vi "Dave_app.vi"() -> ()   [LabVIEW 2015]
uses:
  <vilib>/Utility/file.llb/Write Delimited Spreadsheet (DBL).vi
panel:
  out "Set Value":dbl format="%_6f"
  out "Pcc(uW)":dbl
  out "Vcc(V)":dbl
  out "Icc(uA)":dbl
  in  "Stop":bool
  in  "Export To CSV":bool
  out "Data 2":cluster{dbl[], dbl[]}[](array[cluster])
  out "XY Graph 2":cluster{dbl[], dbl[]}[](graph)
  in  "Voltage Stop (uV)":dbl=0.02
  out "Stop(uA)":dbl
  in  "Load From File":bool
  in  "Save To File":bool
  in  "Clear Last Value":bool
  in  "Clear Graph":bool
  in  "Get Vol":bool
  in  "stop":bool
  out "Data":cluster{dbl[], dbl[]}[](array[cluster])
  in  "VISA resource name":refnum<visa-resource-name>="VAL_N6705B"
  out "XY Graph":cluster{dbl[], dbl[]}[](graph)
  in  "Maker 2 (s)":u16=7
  out "N":u16
  in  "Step(uA)":dbl=10.0
  in  "Start (uA)":dbl min=-1e-05 max=0.0
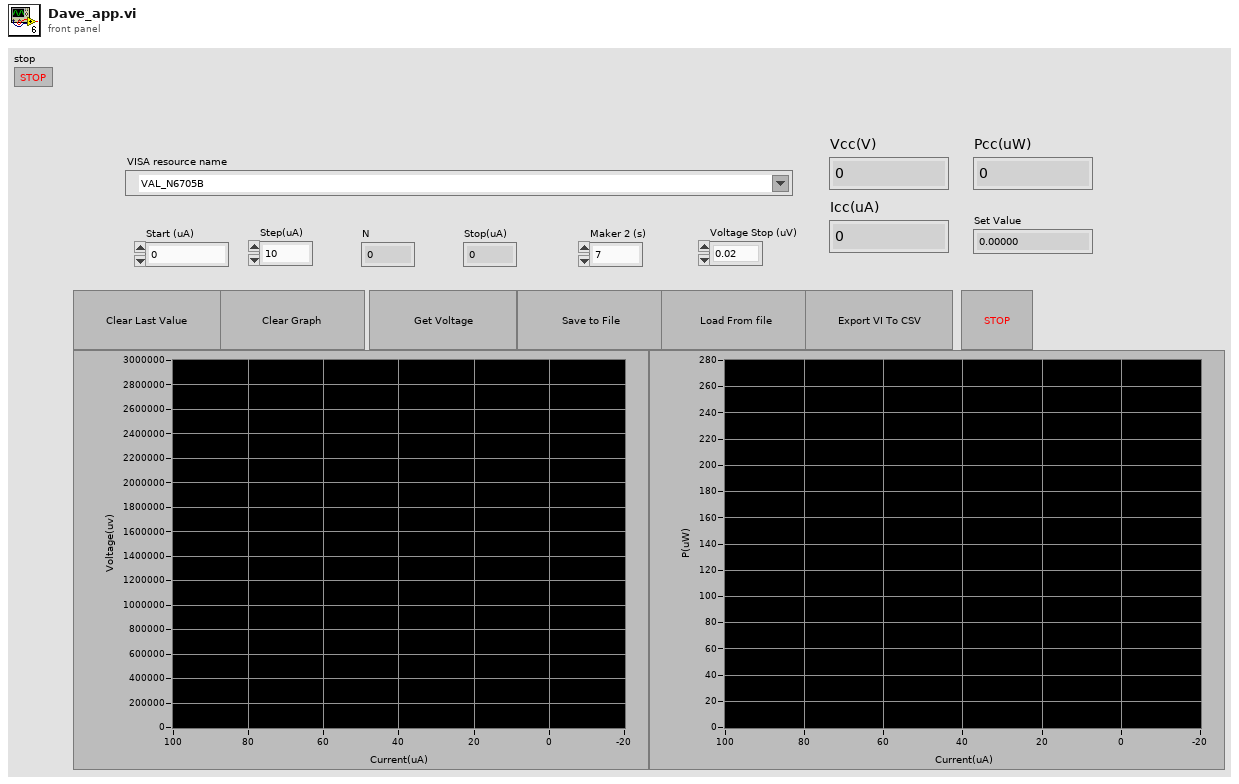
[diagram p1: front panel]
types:
  T1 = enum16{"open", "replace", "create", "open or create", "replace or create", "replace or create with confirmation"}
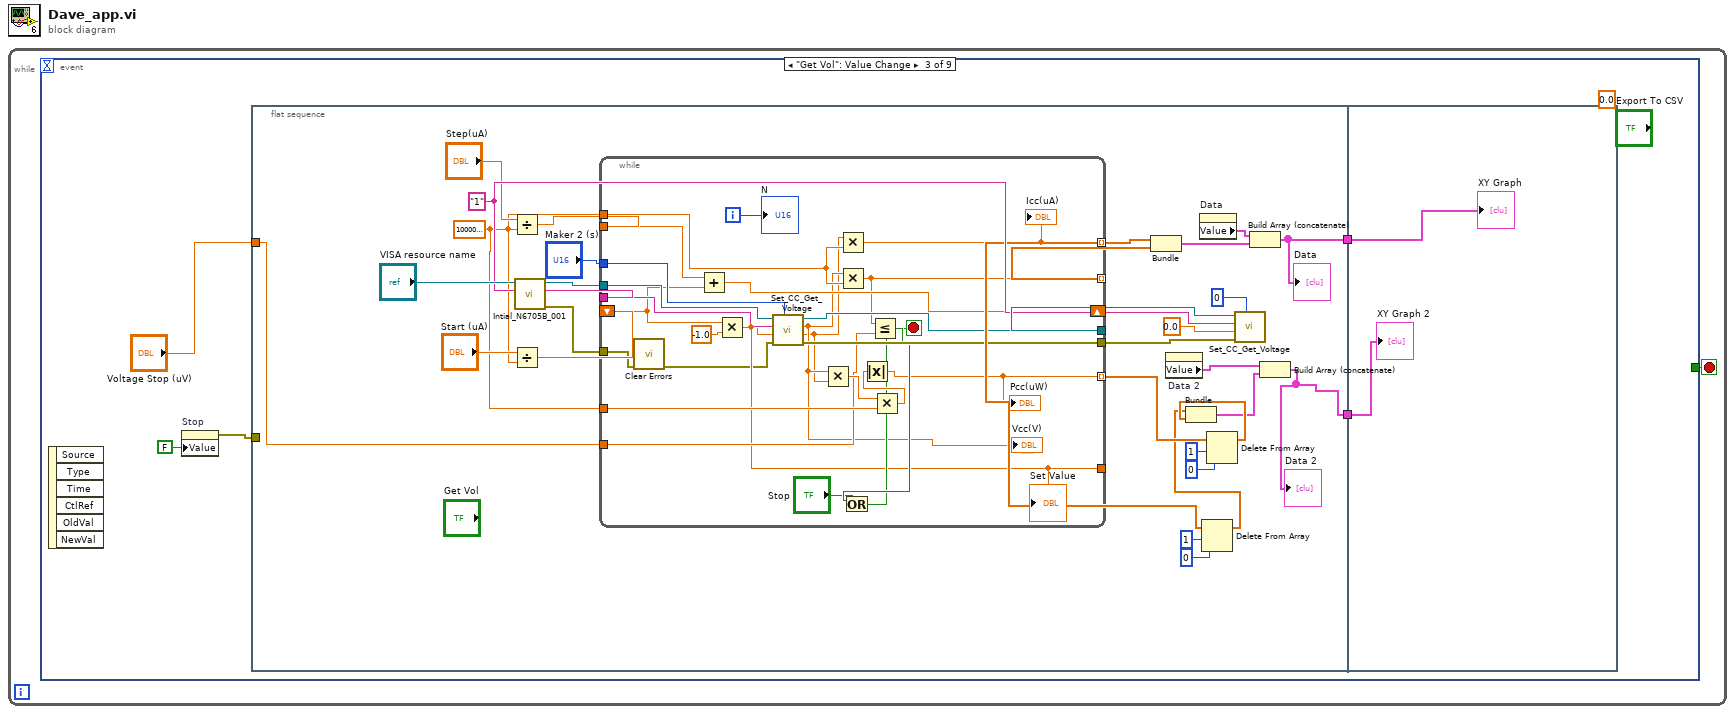
[diagram p0: block diagram]
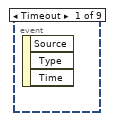
[diagram p2: hidden frame]
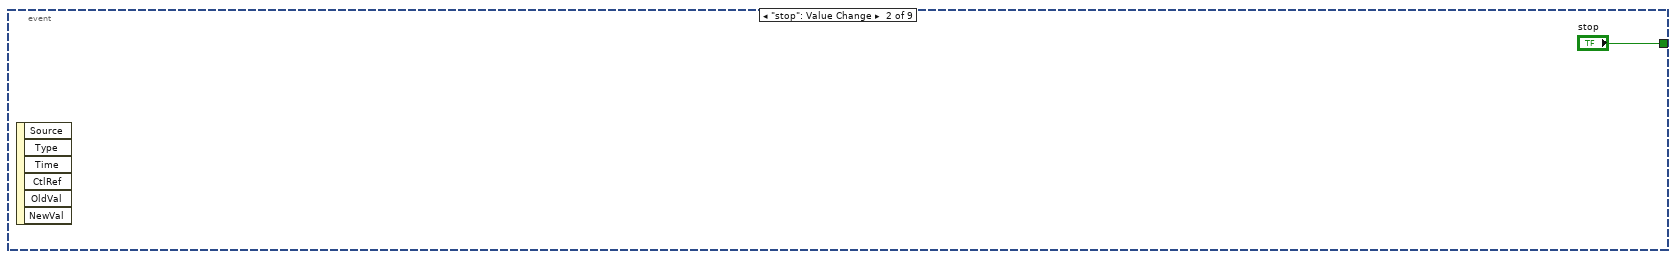
[diagram p3: hidden frame]
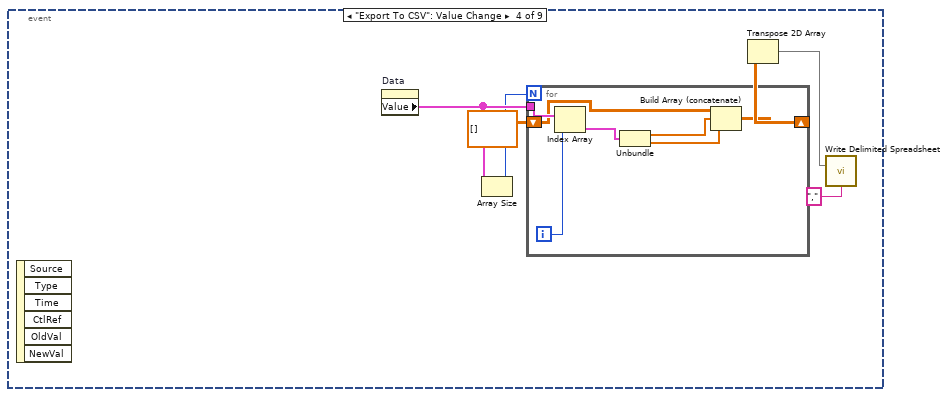
[diagram p4: hidden frame]
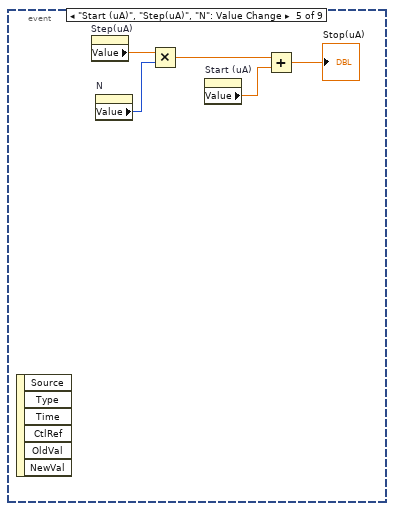
[diagram p5: hidden frame]
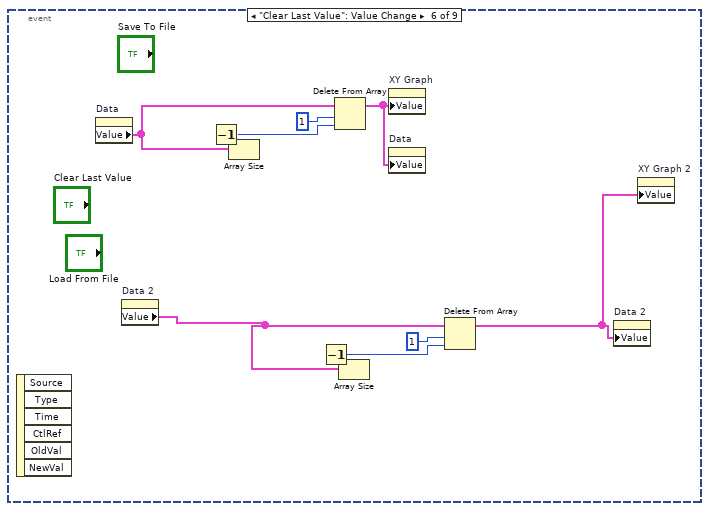
[diagram p6: hidden frame]
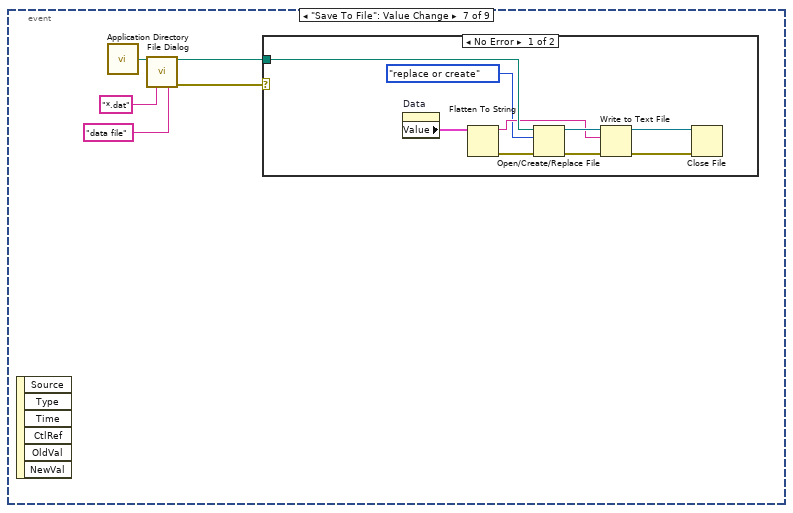
[diagram p7: hidden frame]
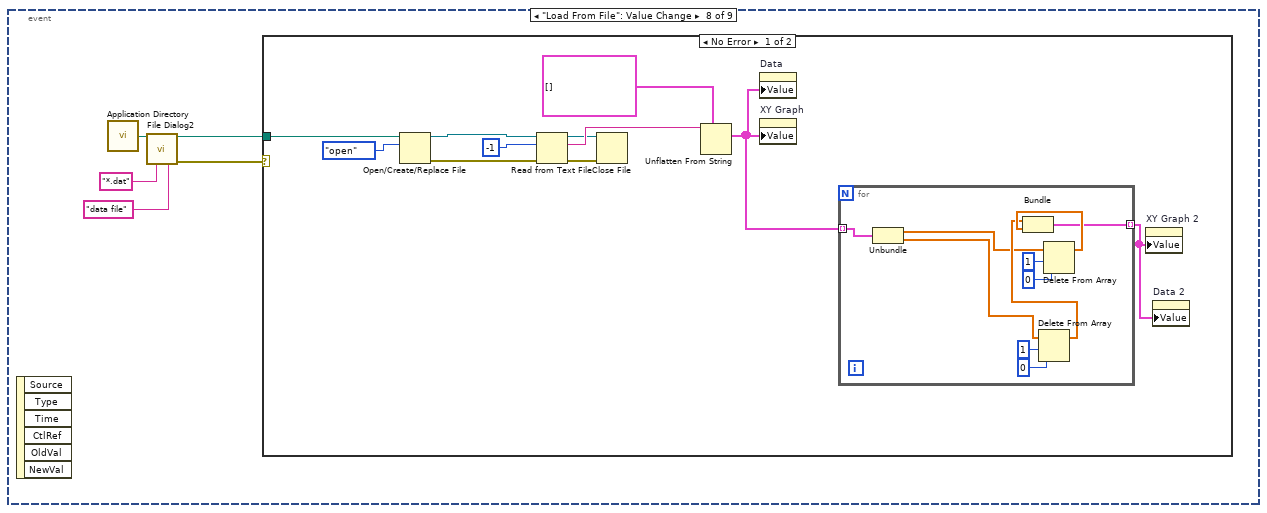
[diagram p9: hidden frame]
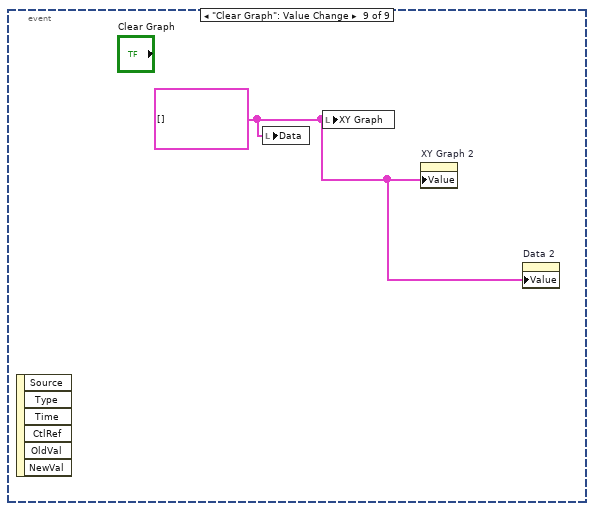
[diagram p11: hidden frame]
diagram:
  n1 = while {
    stop <- w1 stop-if-true
    n2 = event shown="[2] \"Get Vol\": Value Change" {
      selector: _ -> [_ _ _ _ _ _ _ _ _]
      dyn-events: _ -> [_ _ _ _ _ _ _ _ _]
      timeout: _ -> [_ _ _ _ _ _ _ _ _]
      tunnel: [_ "stop" _ _ _ _ _ _ _] -> w1
      event Timeout {
        n3 = event-data() -> ()  [unwired: 1 in, 3 out]
      }
      event "stop": Value Change {
        n4 = event-data() -> ()  [unwired: 1 in, 6 out]
      }
      event "Get Vol": Value Change {
        (unwired) 0.0 ("Scale.Range:Minimum")
        n5 = event-data() -> ()  [unwired: 1 in, 6 out]
        n6 = property on="Stop" class="Bool (strict)"("Value"=FALSE ("Stop")) -> (error out=w3:errorcluster)  [unwired: 2 in, 1 out]
        n7 = flat-sequence {
          tunnel: [w31] -> w7
          tunnel: "Voltage Stop (uV)" -> [w9]
          tunnel: [w11] -> w5
          tunnel: w3 -> [_]
          tunnel: w7 -> [w66]
          tunnel: w5 -> [w65]
          frame #0 {
            w21 = 1000000.0 ("Start (A) 2")
            w27 = "1" ("Channel Name (1)")
            n8 = Divide(x="Step(uA)", y=w21) -> (x/y=w22:dbl)
            n9 = Divide(x="Start (uA)", y=w21) -> (x/y=w24:dbl)
            n10 = call "Intial_N6705B_001.vi"("Channel Name (1) in"=w27, "VISA Refnum in"="VISA resource name") -> ("error out"=w8:errorcluster, "Channel Name (1) out"=w37:string, "VISA Refnum out"=w36:refnum<visa-resource-name>)  [unwired: 7 in]
            n11 = while {
              tunnel: w22 -> [w60]
              tunnel: "Maker 2 (s)" -> [w64]
              tunnel: w36 -> [w63]
              tunnel: w37 -> [w62]
              shift-right: [w61] -> _
              shift-left: w24 -> [w57]
              tunnel: [w54] -> w14 mode=indexing
              tunnel: [w45] -> w38 mode=indexing
              tunnel: [w59] -> w29
              tunnel: [w58] -> w28
              tunnel: w21 -> [w53]
              tunnel: [w43] -> w20 mode=indexing
              tunnel: w21 -> [w51]
              tunnel: w9 -> [w49]
              tunnel: [w42] -> _
              tunnel: w8 -> [w40]
              i -> [w55]
              stop <- w47 stop-if-true
              # "ê"
              n12 = call <vilib>:"Clear Errors.vi"("error in (no error)"=w40) -> ("error out"=w39:errorcluster)  [unwired: 5 in, 1 out]
              n13 = Add(x=w60, y=w57) -> (x+y=w61:dbl)
              n14 = Multiply(x=w57, y=-1.0) -> (x*y=w42:dbl)
              "Set Value" <- w42
              n15 = call "Set_CC_Get_Voltage.vi"("Stop Maker 2"=w64, "error in (no error)"=w39, "Limit (1.0 A)"=w42, "Channel Name (1)"=w62, "VISA Refnum in"=w63) -> ("error out"=w58:errorcluster, "Current Measurement"=w41:dbl, "Voltage Measurement"=w44:dbl, "VISA Refnum out"=w59:refnum<visa-resource-name>)  [unwired: 3 in]
              "Vcc(V)" <- w44
              n16 = Multiply(x=w44, y=w41) -> (x*y=w52:dbl)
              n17 = Multiply(x=w41, y=w53) -> (x*y=w54:dbl)
              "Icc(uA)" <- w54
              n18 = Multiply(x=w44, y=w53) -> (x*y=w45:dbl)
              n19 = Less Or Equal?(x=w45, y=w49) -> (x <= y?=w48:bool)
              n20 = Or(x=w48, y="Stop") -> (x .or. y?=w47:bool)
              n21 = Multiply(x=w52, y=w51) -> (x*y=w50:dbl)
              n22 = Absolute Value(x=w50) -> (abs(x)=w43:dbl)
              "Pcc(uW)" <- w43
              "N" <- w55
            }
            n23 = Bundle(w14, w38) -> (w32:cluster{dbl[], dbl[]})  [unwired: 1 in]
            n24 = property on="Data 2" class="Arr (strict)"() -> ("Value"=w12:cluster{dbl[], dbl[]}[])  [unwired: 2 in, 2 out]
            n25 = property on="Data" class="Arr (strict)"() -> ("Value"=w33:cluster{dbl[], dbl[]}[])  [unwired: 2 in, 2 out]
            n26 = Delete From Array(array=w14, length=1, index=0) -> (array with subset deleted=w13:dbl[])  [unwired: 1 out]
            n27 = Delete From Array(array=w20, length=1, index=0) -> (array with subset deleted=w17:dbl[])  [unwired: 1 out]
            n28 = Bundle(w13, w17) -> (w10:cluster{dbl[], dbl[]})  [unwired: 1 in]
            n29 = call "Set_CC_Get_Voltage.vi"("Stop Maker 2"=u32 0 ("Delay to Measure"), "error in (no error)"=w28, "Limit (1.0 A)"=0.0, "Channel Name (1)"=w27, "VISA Refnum in"=w29) -> ()  [unwired: 3 in, 4 out]
            n30 = Build Array (concatenate)(w33, w32) -> (w31:cluster{dbl[], dbl[]}[])
            "Data" <- w31
            n31 = Build Array (concatenate)(w12, w10) -> (w11:cluster{dbl[], dbl[]}[])
            "Data 2" <- w11
          }
          frame #1 {
            "XY Graph" <- w66
            "XY Graph 2" <- w65
          }
        }
      }
      event "Export To CSV": Value Change {
        n32 = event-data() -> ()  [unwired: 1 in, 6 out]
        n33 = property on="Data" class="Arr (strict)"() -> ("Value"=w69:cluster{dbl[], dbl[]}[])  [unwired: 2 in, 2 out]
        n34 = Array Size(array=w69) -> (size(s)=w68:i32)
        n35 = for {
          N: w68 -> [_]
          tunnel: w69 -> [w75]
          shift-right: [w76] -> w71
          shift-left: dbl[][] [] -> [w73]
          i -> [w74]
          n36 = Index Array(array=w75, index=w74) -> (element=w79:cluster{dbl[], dbl[]})
          n37 = Unbundle(w79) -> (w78:dbl[], w77:dbl[])
          n38 = Build Array (concatenate)(w73, w78, w77) -> (w76:dbl[][])
        }
        n39 = Transpose 2D Array(2D array=w71) -> (transposed array=w70:dbl[][])
        n40 = call-poly <vilib>:"Write Delimited Spreadsheet.vi"("2D data"=w70, "delimiter (\\t)"="," ("delimiter (\\t)")) -> ()  [unwired: 12 in, 2 out]
      }
      event "Start (uA)", "Step(uA)", "N": Value Change {
        n41 = event-data() -> ()  [unwired: 1 in, 6 out]
        n42 = property on="Step(uA)" class="DigNum (strict)"() -> ("Value"=w84:dbl)  [unwired: 2 in, 2 out]
        n43 = property on="N" class="DigNum (strict)"() -> ("Value"=w83:u16)  [unwired: 2 in, 2 out]
        n44 = Multiply(x=w84, y=w83) -> (x*y=w82:dbl)
        n45 = property on="Start (uA)" class="DigNum (strict)"() -> ("Value"=w81:dbl)  [unwired: 2 in, 2 out]
        n46 = Add(x=w82, y=w81) -> (x+y=→"Stop(uA)":dbl)
      }
      event "Clear Last Value": Value Change {
        n47 = event-data() -> ()  [unwired: 1 in, 6 out]
        n48 = property on="Data" class="Arr (strict)"() -> ("Value"=w93:cluster{dbl[], dbl[]}[])  [unwired: 2 in, 2 out]
        n49 = property on="Data 2" class="Arr (strict)"() -> ("Value"=w86:cluster{dbl[], dbl[]}[])  [unwired: 2 in, 2 out]
        n50 = Array Size(array=w93) -> (size(s)=w91:i32)
        n51 = Decrement(x=w91) -> (x-1=w90:i32)
        n52 = Delete From Array(array=w93, length=1, index=w90) -> (array with subset deleted=w92:cluster{dbl[], dbl[]}[])  [unwired: 1 out]
        n53 = Array Size(array=w86) -> (size(s)=w88:i32)
        n54 = Decrement(x=w88) -> (x-1=w89:i32)
        n55 = property on="XY Graph" class="XYGraph (strict)"("Value"=w92) -> ()  [unwired: 2 in, 2 out]
        n56 = property on="Data" class="Arr (strict)"("Value"=w92) -> ()  [unwired: 2 in, 2 out]
        n57 = Delete From Array(array=w86, length=1, index=w89) -> (array with subset deleted=w85:cluster{dbl[], dbl[]}[])  [unwired: 1 out]
        n58 = property on="Data 2" class="Arr (strict)"("Value"=w85) -> ()  [unwired: 2 in, 2 out]
        n59 = property on="XY Graph 2" class="XYGraph (strict)"("Value"=w85) -> ()  [unwired: 2 in, 2 out]
      }
      event "Save To File": Value Change {
        n60 = event-data() -> ()  [unwired: 1 in, 6 out]
        n61 = call <vilib>:"Application Directory.vi"() -> ("Application Directory"=w99:path)
        n62 = call "File Dialog"("start path"=w99, "pattern (all files)"="*.dat", "pattern label"="data file") -> ("selected path"=w96:path, "error out"=w95:errorcluster)  [unwired: 9 in, 2 out]
        n63 = case shown="No Error" w95 {
          tunnel: w96 -> [w107 _]
          frame No Error {
            n64 = property on="Data" class="Arr (strict)"() -> ("Value"=w108:cluster{dbl[], dbl[]}[])  [unwired: 2 in, 2 out]
            n65 = Flatten To String(anything=w108) -> (data string=w105:string, error out=w104:errorcluster)  [unwired: 3 in, 1 out]
            n66 = Open/Create/Replace File(file path (use dialog)=w107, error in=w104, operation (0:open)=T1."replace or create") -> (refnum out=w106:refnum<file>, error out=w103:errorcluster)  [unwired: 3 in, 1 out]
            n67 = Write to Text File(file (use dialog)=w106, text=w105, error in=w103) -> (refnum out=w102:refnum<file>, error out=w101:errorcluster)  [unwired: 1 in, 1 out]
            n68 = Close File(refnum=w102, error in=w101) -> ()  [unwired: 2 out]
          }
          frame Error {
          }
        }
      }
      event "Load From File": Value Change {
        n69 = event-data() -> ()  [unwired: 1 in, 6 out]
        n70 = call <vilib>:"Application Directory.vi"() -> ("Application Directory"=w113:path)
        n71 = call "File Dialog2"("start path"=w113, "pattern (all files)"="*.dat", "pattern label"="data file") -> ("selected path"=w110:path, "error out"=w109:errorcluster)  [unwired: 9 in, 2 out]
        n72 = case shown="No Error" w109 {
          tunnel: w110 -> [w124 _]
          frame No Error {
            n73 = Open/Create/Replace File(file path (use dialog)=w124, operation (0:open)=T1."open") -> (refnum out=w122:refnum<file>, error out=w120:errorcluster)  [unwired: 4 in, 1 out]
            n74 = Read from Text File(file (use dialog)=w122, count=-1, error in=w120) -> (refnum out=w117:refnum<file>, text=w119:string, error out=w116:errorcluster)  [unwired: 1 in, 1 out]
            n75 = Close File(refnum=w117, error in=w116) -> ()  [unwired: 2 out]
            n76 = Unflatten From String(type=cluster{dbl[], dbl[]}[] [] ("Data"), binary string=w119) -> (value=w115:cluster{dbl[], dbl[]}[])  [unwired: 3 in, 2 out]
            n77 = property on="Data" class="Arr (strict)"("Value"=w115) -> ()  [unwired: 2 in, 2 out]
            n78 = property on="XY Graph" class="XYGraph (strict)"("Value"=w115) -> ()  [unwired: 2 in, 2 out]
            n79 = for {
              tunnel: w115 -> [w134] mode=indexing
              tunnel: [w125] -> w114 mode=indexing
              n80 = Unbundle(w134) -> (w127:dbl[], w126:dbl[])
              n81 = Delete From Array(array=w126, length=1, index=0) -> (array with subset deleted=w128:dbl[])  [unwired: 1 out]
              n82 = Delete From Array(array=w127, length=1, index=0) -> (array with subset deleted=w131:dbl[])  [unwired: 1 out]
              n83 = Bundle(w128, w131) -> (w125:cluster{dbl[], dbl[]})  [unwired: 1 in]
            }
            n84 = property on="XY Graph 2" class="XYGraph (strict)"("Value"=w114) -> ()  [unwired: 2 in, 2 out]
            n85 = property on="Data 2" class="Arr (strict)"("Value"=w114) -> ()  [unwired: 2 in, 2 out]
          }
          frame Error {
          }
        }
      }
      event "Clear Graph": Value Change {
        w135 = cluster{dbl[], dbl[]}[] [] ("XY Graph")
        n86 = event-data() -> ()  [unwired: 1 in, 6 out]
        n87 = local write "Data"(w135) -> ()
        n88 = local write "XY Graph"(w135) -> ()
        n89 = property on="XY Graph 2" class="XYGraph (strict)"("Value"=w135) -> ()  [unwired: 2 in, 2 out]
        n90 = property on="Data 2" class="Arr (strict)"("Value"=w135) -> ()  [unwired: 2 in, 2 out]
      }
    }
  }
